vi "array -- bilinear regression 2D -- curvature wrapper -- V2.vi"(7 "action":T6, 8 "2D curvature tensor IN":T2={"curvature Matrix"=[[3.0, 1.0], [1.0, 4.0]], "eigenvs"=[4.618033988749895, 2.381966011250105], "Eigenvectors"=[[-0.8506508083520399+0.0i, -0.5257311121191335+0.0i], [0.5257311121191335+0.0i, -0.8506508083520399+0.0i]], "theta (rad)"=0.5535743588970453, "theta (deg)"=31.717474411461012, "Δs"=[4.618033988749895, 2.381966011250105], "δG/G"=0.5535743588970453, "δs"=[4.618033988749895, 2.381966011250105], "inverse Matrix"=[[3.0, 1.0], [1.0, 4.0]], "noise T"=0.5535743588970453, "pars & errors"={}} {"noise T" format="%#_3p"; "inverse Matrix" format="%#_3p"; "δs" format="%#_2p"; "δG/G" format="%#_3p"; "Δs" format="%#_3p"; "theta (deg)" format="%#_3p"; "curvature Matrix" format="%#_3p"; "eigenvs" format="%#_3p"; "Eigenvectors" format="%#_3p"; "theta (rad)" format="%#_3p"}, 9 "fit map IN":map{T1, dbl}(c390)={enum."1"=0.0, enum."x"=0.0, enum."y"=0.0, enum."xx"=1.0, enum."xy"=1.0, enum."yy"=1.0}, 11 "xyz IN":cluster{"x":dbl[], "y":dbl[], "z":dbl[]}={"x"=[10.0, -7.0, 6.0, -1.0, -1.0, -1.0, 1.0, 1.0], "y"=[-1.0, 4.0, 45.0, -1.0, -23.0, 1.0, -1.0, 2.0], "z"=[1.0, -5.0, 1.0, 4.0, 1.0, 43.0, -4.0, 12.0]}) -> (0 "2D curvature tensor OUT":T2={"curvature Matrix"=[[0.9999999999999996, 0.9999999999999998], [0.9999999999999998, 1.0]], "eigenvs"=[1.7838428397948585, 0.21615716020514097], "Eigenvectors"=[[-0.8506508083520399+0.0i, -0.5257311121191335+0.0i], [0.5257311121191335+0.0i, -0.8506508083520399+0.0i]], "theta (rad)"=0.7853981633974482, "theta (deg)"=44.99999999999999, "Δs"=[nan, nan], "δG/G"=0.5535743588970453, "δs"=[4.618033988749895, 2.381966011250105], "inverse Matrix"=[], "noise T"=0.5535743588970453, "pars & errors"={}} {"noise T" format="%#_3p"; "inverse Matrix" format="%#_3p"; "δs" format="%#_2p"; "δG/G" format="%#_3p"; "Δs" format="%#_3p"; "theta (deg)" format="%#_3p"; "curvature Matrix" format="%#_3p"; "eigenvs" format="%#_3p"; "Eigenvectors" format="%#_3p"; "theta (rad)" format="%#_3p"}, 1 "fit map out":map{T1, dbl}(c390)={enum."1"=0.0, enum."x"=0.0, enum."y"=1.1102230246251565e-16, enum."xx"=0.9999999999999996, enum."xy"=0.9999999999999998, enum."yy"=1.0}, 3 "xyz OUT":cluster{"x":dbl[], "y":dbl[], "z":dbl[]}={"x"=[0.0, 0.0, 0.0, -1.0, -1.0, -1.0, 1.0, 1.0], "y"=[-1.0, 0.0, 1.0, -1.0, 0.0, 1.0, -1.0, 0.0], "z"=[1.0, 0.0, 1.0, 4.0, 1.0, 0.0, 0.0, 1.0]})   [LabVIEW 2021]
uses:
  array -- fit control .ctl
  array -- bilinear regression 2D.ctl
  <vilib>/Analysis/Matrix/Datatypes/RealMatrix.ctl
  2D curvature tensor.ctl
  <vilib>/Analysis/Matrix/Datatypes/ComplexMatrix.ctl
  3-lorentzian-parameters.ctl
  2D curvature tensor actions.ctl
  <vilib>/Analysis/baseanly.llb/A x B.vi
  <vilib>/Analysis/baseanly.llb/Real A x B.vi
  <vilib>/Analysis/Matrix/Numeric/Conversions/Array To Matrix - RA2.vi
  <vilib>/Analysis/baseanly.llb/Inverse Matrix.vi
  <vilib>/Analysis/baseanly.llb/Real Inverse Matrix.vi
  <vilib>/Analysis/Matrix/Numeric/Conversions/Matrix To Array.vi
  <vilib>/Analysis/Matrix/Numeric/Conversions/Matrix To Array - RM.vi
  <vilib>/Analysis/Matrix/NI_Matrix.lvlib
panel:
  out "curvature Matrix":T3=[[0.9999999999999996, 0.9999999999999998], [0.9999999999999998, 1.0]]
  out "y OUT":dbl[](array[numeric])=[-1.0, 0.0, 1.0, -1.0, 0.0, 1.0, -1.0, 0.0]
  out "y":dbl[](array[numeric])=[-1.0, 0.0, 1.0, -1.0, 0.0, 1.0, -1.0, 0.0]
  out "x OUT":dbl[](array[numeric])=[0.0, 0.0, 0.0, -1.0, -1.0, -1.0, 1.0, 1.0]
  out "z OUT":dbl[](array[numeric])=[1.0, 0.0, 1.0, 4.0, 1.0, 0.0, 0.0, 1.0]
  out "fit  IN":dbl[](array[numeric])=[1.0, 1.0, 1.0, 0.0, 0.0, 0.0]
  out "fit OUT":dbl[](array[numeric])=[0.9999999999999996, 0.9999999999999998, 1.0, 0.0, 1.1102230246251565e-16, 0.0]
  out "z":dbl[](array[numeric])=[1.0, 0.0, 1.0, 4.0, 1.0, 0.0, 0.0, 1.0]
  out "x":dbl[](array[numeric])=[0.0, 0.0, 0.0, -1.0, -1.0, -1.0, 1.0, 1.0]
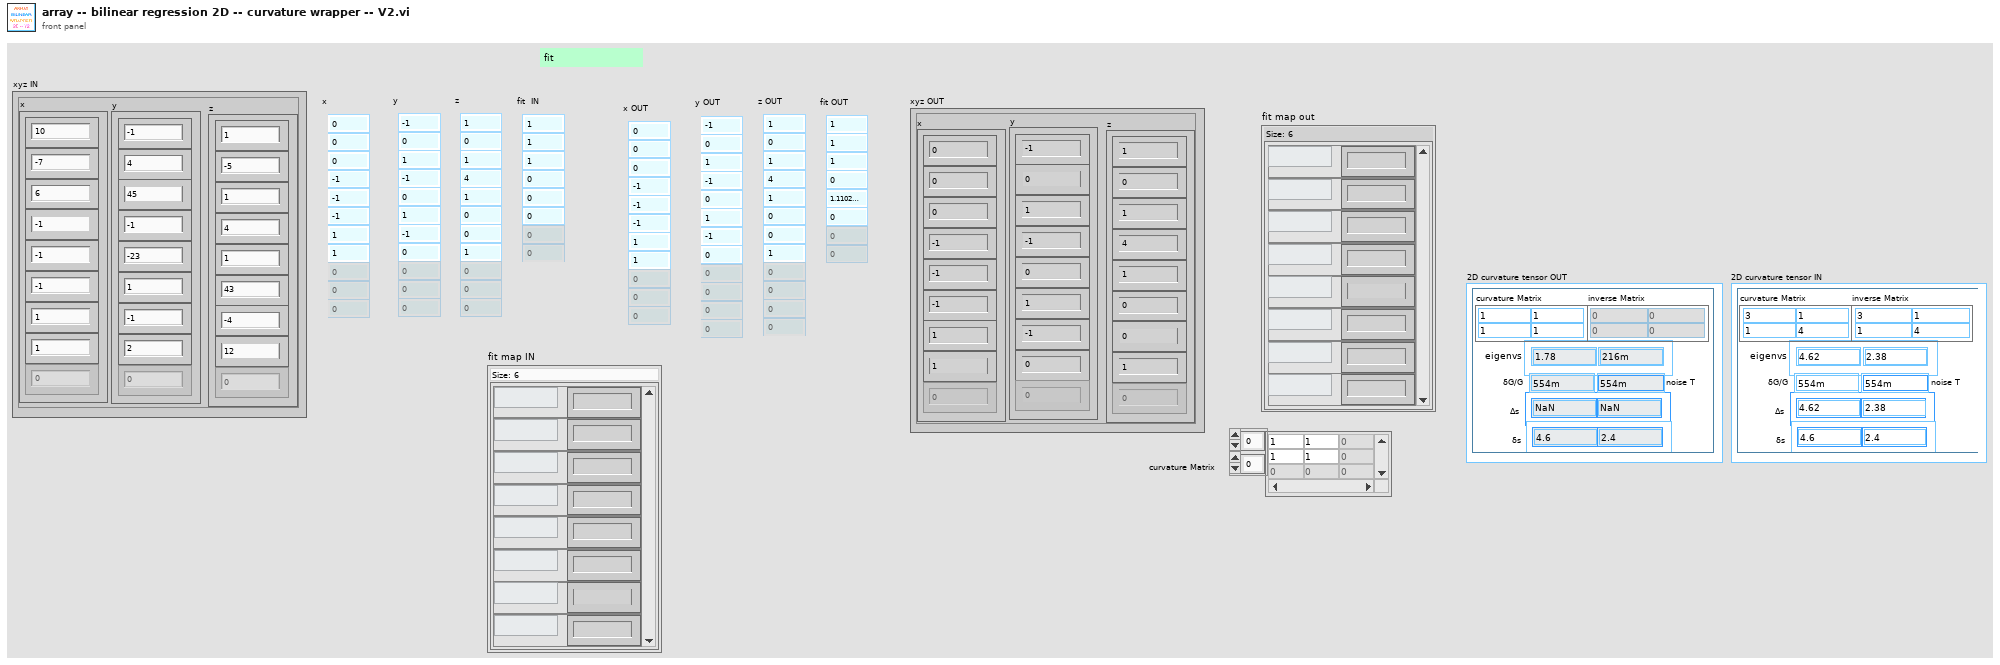
[diagram p1: front panel]
types:
  T1 = typedef "array -- bilinear regression 2D.ctl" = enum16{"1", "x", "y", "xx", "xy", "yy", "xxy", "xyy", "yyy", "xxx", "xxyy", "xyyy", "xxxy", "yyyy", "xxxx", "xxz", "xyz", "yyz", "xz", "yz", "z"}
  T2 = typedef "2D curvature tensor.ctl" = cluster{"curvature Matrix":T3, "eigenvs":dbl[], "Eigenvectors":T4, "theta (rad)":dbl, "theta (deg)":dbl, "Δs":dbl[], "δG/G":dbl, "δs":dbl[], "inverse Matrix":T3, "noise T":dbl, "pars & errors":map{T5, dbl}}
  T3 = typedef "NI_Matrix.lvlib/RealMatrix.ctl" = dbl[][]
  T4 = typedef "NI_Matrix.lvlib/ComplexMatrix.ctl" = cdb[][]
  T5 = typedef "3-lorentzian-parameters.ctl" = enum16{"ζ", "τ1", "τS", "τN", "τC", "κ0", "m1", "m2", "m3", "T (K)", "B (T)", "θ (deg)", "side (S|R)", "set of (B|T)", "Re(offset)", "Im(offset)", "στ1", "στ1-", "στ1+", "στS", "στS-", "στS+", "στN", "στN-", "στN+"}
  T6 = typedef "array -- fit control .ctl" = enum16{"fit", "calc", "check", "init"}
  T7 = typedef "2D curvature tensor actions.ctl" = enum16{"eigensystem", "sigma", "set matrix", "inverse"}
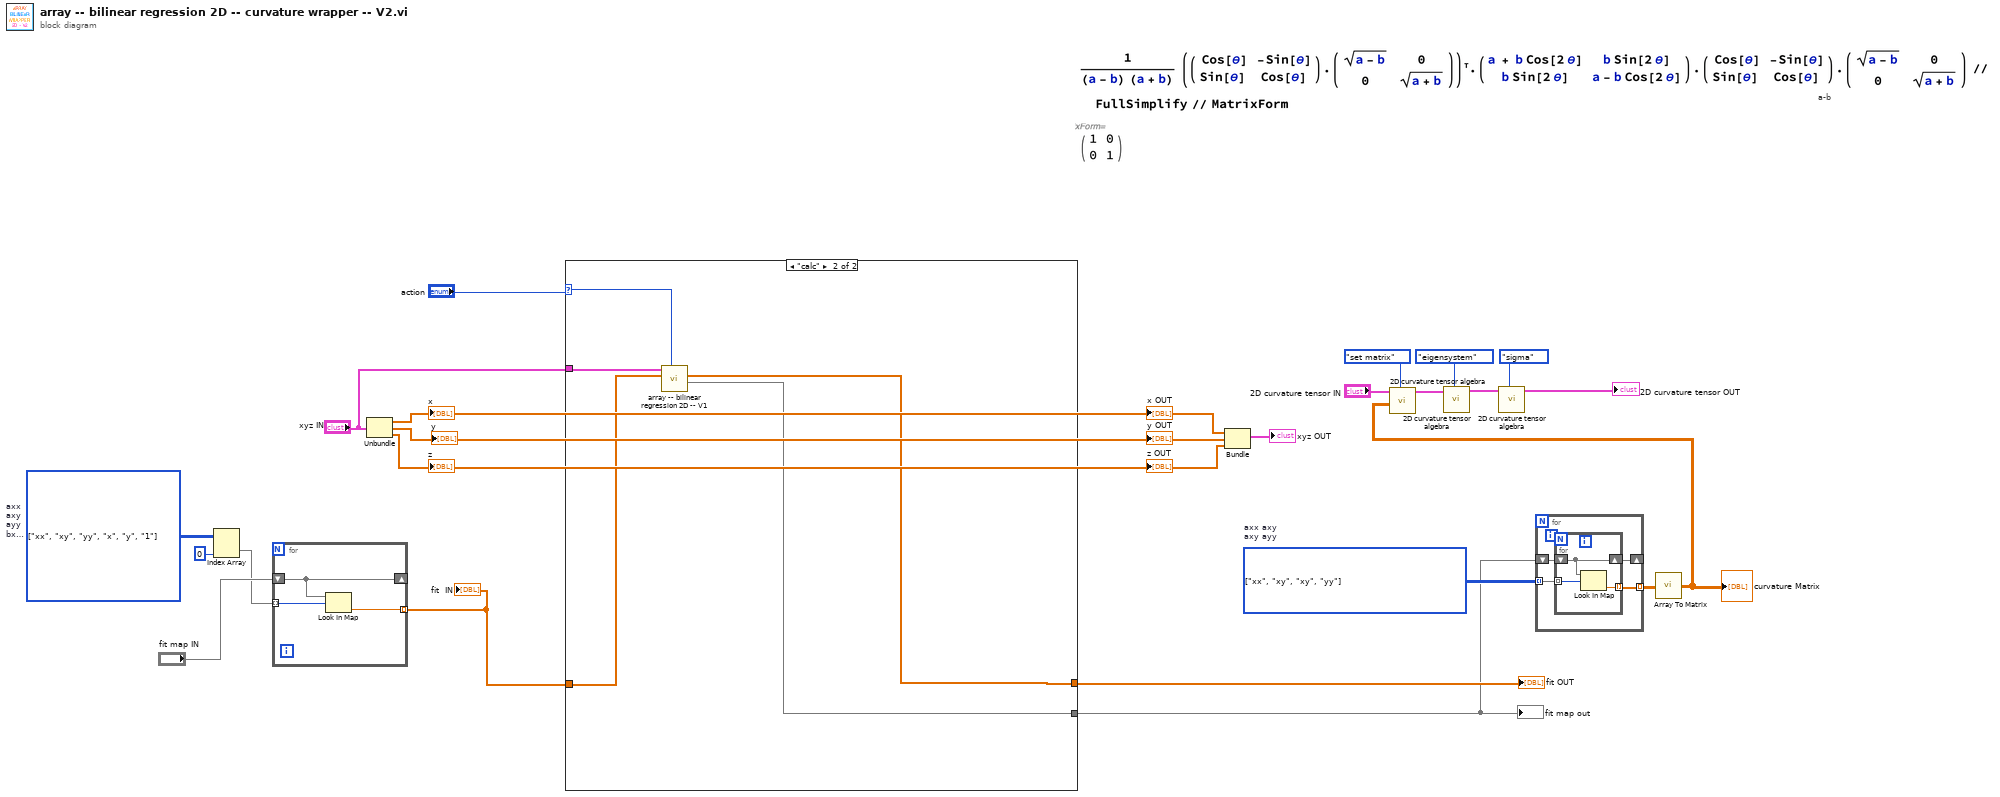
[diagram p0: block diagram]
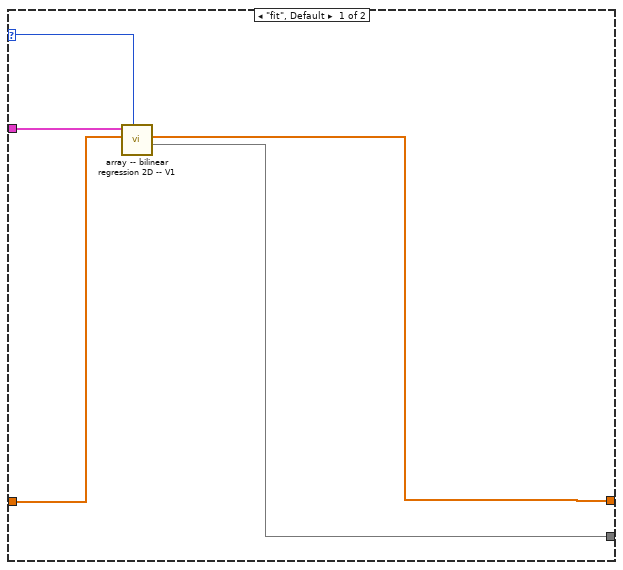
[diagram p2: hidden frame]
diagram:
  w5 = T1[][] [[enum."xx"], [enum."xy"], [enum."yy"], [enum."x"], [enum."y"], [enum."1"]] items=["1", "x", "y", "xx", "xy", "yy", "xxy", "xyy", "yyy", "xxx", "xxyy", "xyyy", "xxxy", "yyyy", "xxxx", "xxz", "xyz", "yyz", "xz", "yz", "z"]  # axx axy ayy bx by c
  w21 = T1[][] [[enum."xx", enum."xy"], [enum."xy", enum."yy"]] items=["1", "x", "y", "xx", "xy", "yy", "xxy", "xyy", "yyy", "xxx", "xxyy", "xyyy", "xxxy", "yyyy", "xxxx", "xxz", "xyz", "yyz", "xz", "yz", "z"]  # axx axy axy ayy
  # "a-b"
  n1 = Index Array(array=w5, index (col)=0 ("disabled index (col)")) -> (element=w2:T1[])  [unwired: 1 in]
  n2 = for {
    shift-right: [w24] -> _
    shift-left: "fit map IN" -> [w24]
    tunnel: w2 -> [w26] mode=indexing
    tunnel: [w25] -> w1 mode=indexing
    n3 = Look In Map(map=w24, key=w26) -> (value=w25:dbl)  [unwired: 1 in, 1 out]
  }
  "fit  IN" <- w1
  n4 = Unbundle("xyz IN") -> ("x"=w12:dbl[], "y"=w11:dbl[], "z"=w10:dbl[])
  "x" <- w12
  "z" <- w10
  "z OUT" <- w10
  "x OUT" <- w12
  "y OUT" <- w11
  "y" <- w11
  n5 = case shown="\"calc\"" "action" {
    selector: "action" -> [w28 w33]
    tunnel: "xyz IN" -> [w31 w36]
    tunnel: [w30 w35] -> w8
    tunnel: [w29 w34] -> w7
    tunnel: w1 -> [w27 w32]
    frame "fit", Default {
      n6 = call "array -- bilinear regression 2D -- V1.vi"("action"=w28, "fit  IN"=w27, "xyz IN"=w31) -> ("fit map out"=w29:map{T1, dbl}, "fit OUT"=w30:dbl[])  [unwired: 6 in, 1 out]
    }
    frame "calc" {
      n7 = call "array -- bilinear regression 2D -- V1.vi"("action"=w33, "fit  IN"=w32, "xyz IN"=w36) -> ("fit map out"=w34:map{T1, dbl}, "fit OUT"=w35:dbl[])  [unwired: 6 in, 1 out]
    }
  }
  "fit OUT" <- w8
  "fit map out" <- w7
  n8 = Bundle("x"=w12, "y"=w11, "z"=w10) -> (→"xyz OUT":cluster{"x":dbl[], "y":dbl[], "z":dbl[]})  [unwired: 1 in]
  n9 = for {
    tunnel: w21 -> [w40] mode=indexing
    shift-right: [w38] -> _
    shift-left: w7 -> [w39]
    tunnel: [w37] -> w22 mode=indexing
    n10 = for {
      tunnel: w40 -> [w42] mode=indexing
      shift-right: [w43] -> w38
      shift-left: w39 -> [w43]
      tunnel: [w41] -> w37 mode=indexing
      n11 = Look In Map(map=w43, key=w42) -> (value=w41:dbl)  [unwired: 1 in, 1 out]
    }
  }
  n12 = call-poly <vilib>:"Array To Matrix.vi"("Real 2D Array"=w22) -> ("Real Matrix"=w17:T3)
  "curvature Matrix" <- w17
  n13 = call "2D curvature tensor algebra.vi"("2D tensor"=2D_curvature_tensor_actions."set matrix", "2D curvature Matrix IN"=w17, "curvature tensor IN"="2D curvature tensor IN") -> ("curvature tensor OUT"=w19:T2)  [unwired: 7 in, 1 out]
  n14 = call "2D curvature tensor algebra.vi"("2D tensor"=2D_curvature_tensor_actions."eigensystem", "curvature tensor IN"=w19) -> ("curvature tensor OUT"=w16:T2)  [unwired: 8 in, 1 out]
  n15 = call "2D curvature tensor algebra.vi"("2D tensor"=2D_curvature_tensor_actions."sigma", "curvature tensor IN"=w16) -> ("curvature tensor OUT"=→"2D curvature tensor OUT":T2)  [unwired: 8 in, 1 out]
